vi "Append log file (create path and file as needed).vi"(8 "error in":errorcluster, 10 "text to append":string, 11 "Log file path":string) -> (0 "error out":errorcluster, 3 "Log string":string)   [LabVIEW 2013]
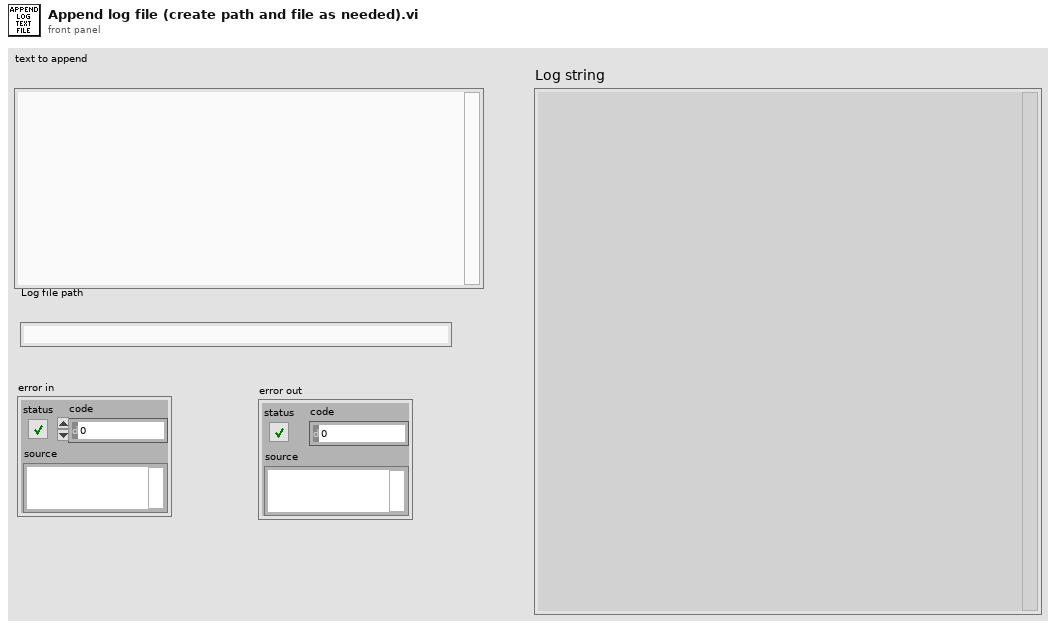
[diagram p1: front panel]
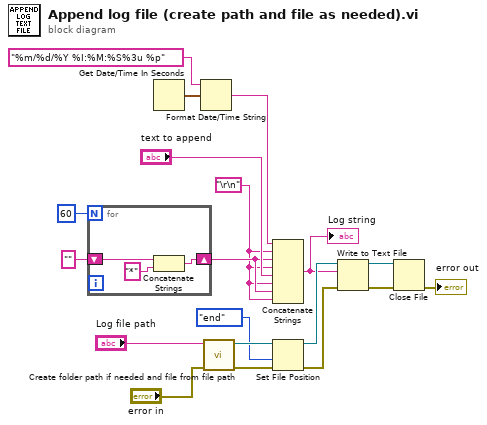
[diagram p0: block diagram]
diagram:
  w4 = "\r\n"
  n1 = for {
    N: 60 -> [_]
    shift-right: [w20] -> w5
    shift-left: "" -> [w22]
    n2 = Concatenate Strings(w22, "*" ("string")) -> (w20:string)
  }
  n3 = Get Date/Time In Seconds() -> (seconds since 1Jan1904=w3:timestamp)
  n4 = Format Date/Time String(time format string (%c)="%m/%d/%Y %I:%M:%S%3u %p", seconds (now)=w3) -> (date/time string=w1:string)  [unwired: 1 in]
  n5 = call "Create folder path if needed and file from file path.vi"("error in"="error in", "String file path"="Log file path") -> ("error out"=w15:errorcluster, "New file refnum"=w17:refnum<file>)  [unwired: 7 in, 1 out]
  n6 = Concatenate Strings(w1, w4, w5, w4, "text to append", w4, w5, w4) -> (w11:string)
  "Log string" <- w11
  n7 = Set File Position(refnum=w17, from (0:start)=enum16{"start", "end", "current"}."end", error in=w15) -> (refnum out=w14:refnum<file>, error out=w13:errorcluster)  [unwired: 1 in]
  n8 = Write to Text File(file (use dialog)=w14, text=w11, error in=w13) -> (refnum out=w9:refnum<file>, error out=w10:errorcluster)  [unwired: 1 in, 1 out]
  n9 = Close File(refnum=w9, error in=w10) -> (error out=→"error out":errorcluster)  [unwired: 1 out]
